vi "Close.vi"   [LabVIEW 2020, in "nisyscfg.lvlib"]
doc: "Closes a reference to a previously allocated filter, resource, or session. Error I/O operates uniquely in this function. The function closes the device session regardless of whether an error occurred in a preceding operation."
uses:
  <vilib>/nisyscfg/nisyscfg.lvlib
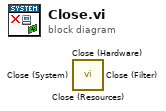
[diagram p0: block diagram]
diagram:
  n1 = call <vilib>:"Close (Resources).vi"() -> ()  [unwired: 11 in, 1 out]
  n2 = call <vilib>:"Close (Hardware).vi"() -> ()  [unwired: 11 in, 1 out]
  n3 = call <vilib>:"Close (System).vi"() -> ()  [unwired: 11 in, 1 out]
  n4 = call <vilib>:"Close (Filter).vi"() -> ()  [unwired: 11 in, 1 out]
